vi "Stop gRPC Server.vi"(8 "error in (no error)":errorcluster, 11 "CIFCorePlugin in":refnum<class "CIFCorePlugin.lvclass">) -> (0 "error out":errorcluster, 3 "CIFCorePlugin out":refnum<class "CIFCorePlugin.lvclass">)   [LabVIEW 2021, in "CIFCorePlugin.lvclass"]
uses:
  CIFCorePlugin.lvclass
  CIFCorePlugin.lvclass/CIFCorePlugin.ctl
  CIFCoreGrpc/CIFCorePlugin_server/RPC Service/PluginCore/PluginCore.lvclass
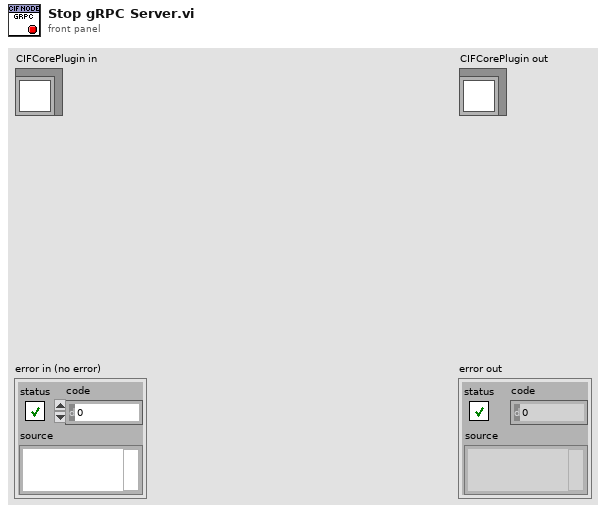
[diagram p1: front panel]
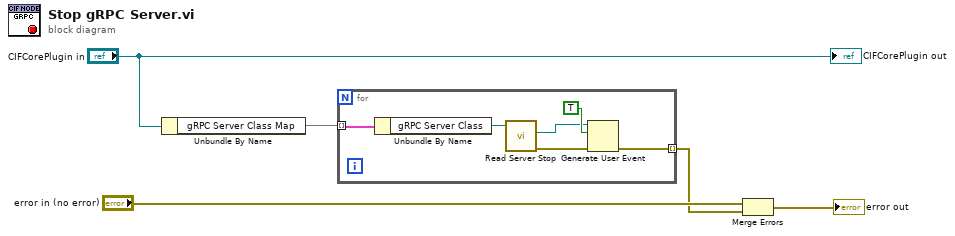
[diagram p0: block diagram]
diagram:
  n1 = Unbundle By Name("CIFCorePlugin in") -> ("gRPC Server Class Map"=w4:map{string, refnum<class "PluginCore.lvclass">})
  n2 = for {
    tunnel: w4 -> [w8] mode=indexing
    tunnel: [w6] -> w2 mode=indexing
    n3 = Unbundle By Name(w8) -> ("gRPC Server Class"=w7:refnum<class "PluginCore.lvclass">)
    n4 = call-dynamic "Read Server Stop.vi"("iService in"=w7) -> ("error out"=w9:errorcluster, "Server Stop"=w10:refnum<user-event>)  [unwired: 8 in, 1 out]
    n5 = Generate User Event(user event=w10, event data cluster=TRUE, error in=w9) -> (error out=w6:errorcluster)  [unwired: 1 in, 1 out]
  }
  n6 = Merge Errors("error in (no error)", w2) -> (→"error out":errorcluster)
  "CIFCorePlugin out" <- "CIFCorePlugin in"
